vi "read files to include.vi"(11 "Builder in":refnum<class "Builder.lvclass">) -> (2 "files to include":string[](array[string]))   [LabVIEW 2024, in "Builder.lvclass"]
uses:
  Builder.lvclass
  Builder.lvclass/Builder.ctl
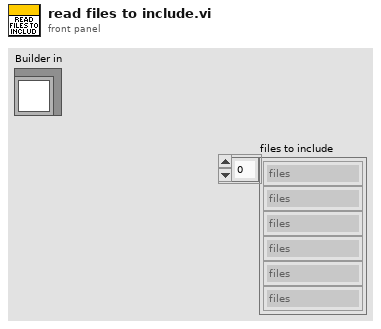
[diagram p1: front panel]
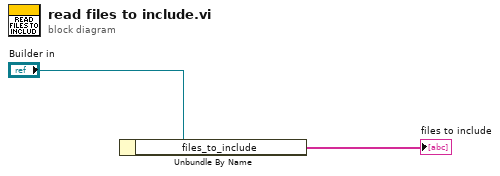
[diagram p0: block diagram]
diagram:
  n1 = Unbundle By Name("Builder in") -> ("files_to_include"=→"files to include":string[])
